vi "readStart.vi"(8 "error in (no error)":errorcluster, 11 "ElectrometerReadingStatus in":refnum<class "ElectrometerReadingStatus.lvclass">) -> (0 "error out":errorcluster, 3 "ElectrometerReadingStatus out":refnum<class "ElectrometerReadingStatus.lvclass">)   [LabVIEW 2016, in "ElectrometerReadingStatus.lvclass"]
uses:
  ElectrometerReadingStatus.lvclass
  ElectrometerReadingVar.vi
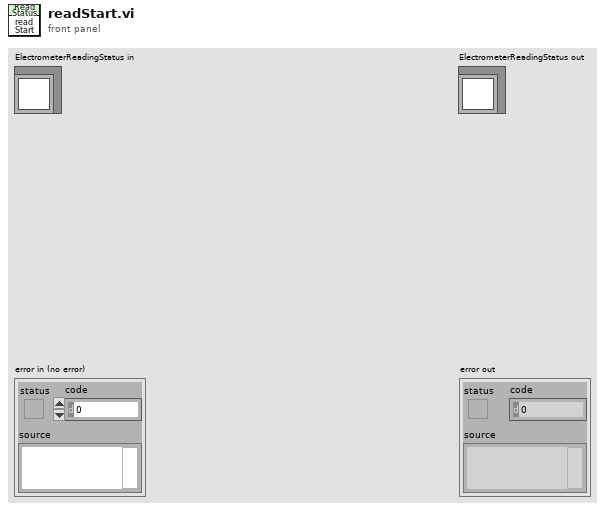
[diagram p1: front panel]
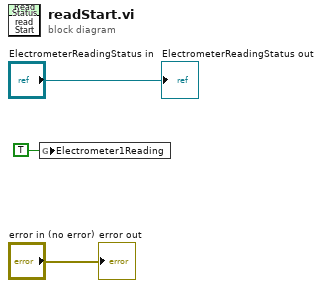
[diagram p0: block diagram]
diagram:
  n1 = global write "ElectrometerReadingVar.vi" "Electrometer1Reading"(TRUE ("Electrometer1Reading")) -> ()
  "error out" <- "error in (no error)"
  "ElectrometerReadingStatus out" <- "ElectrometerReadingStatus in"
